vi "SynapseAPI-Set Block (unique).vi"(0 "URL":string="http://localhost:24414", 7 "block":string, 11 "error in (no error)":errorcluster) -> (15 "error out":errorcluster)   [LabVIEW 2020]
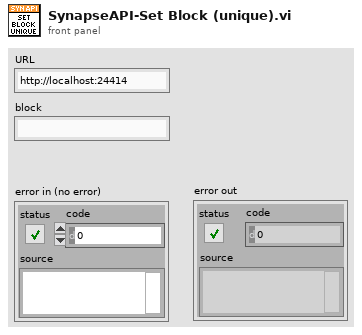
[diagram p1: front panel]
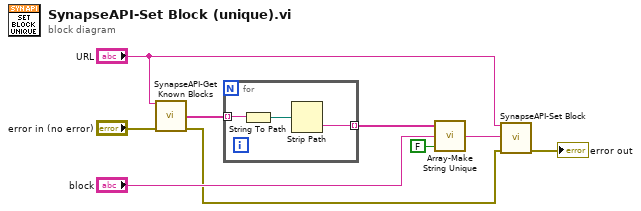
[diagram p0: block diagram]
diagram:
  n1 = call "SynapseAPI-Get Known Blocks.vi"("URL"="URL", "error in (no error)"="error in (no error)") -> ("blocks"=w3:string[], "error out"=w6:errorcluster)  [unwired: 12 in]
  n2 = for {
    tunnel: w3 -> [w12] mode=indexing
    tunnel: [w10] -> w2 mode=indexing
    n3 = String To Path(string=w12) -> (path=w11:path)
    n4 = Strip Path(path=w11) -> (name=w10:string)  [unwired: 1 out]
  }
  n5 = call "Array-Make String Unique.vi"("Use parentheses"=FALSE, "String"="block", "Strings"=w2) -> ("Unique String"=w7:string)  [unwired: 2 in]
  n6 = call "SynapseAPI-Set Block.vi"("URL"="URL", "block"=w7, "error in (no error)"=w6) -> ("error out"=→"error out":errorcluster)  [unwired: 12 in]
